vi "Labview_code_used_in_serum_and_PBS_experiments.vi"() -> ()   [LabVIEW 2018]
doc: "Example: Stream to Disk\n\nRecommended Input Signal: 100kHz, 2Vpp, sine wave\n\nDevices Supported: Refer to NI Example Finder\n\nLabVIEW Description:\n\nThis example demonstrates streaming a continuous acquisition to disk. It configures and starts one acquisition that is never triggered. This is accomplished by configuring a software trigger and never sending the software trigger. Therefore, the digitizer will continuously acquire data into its onboard memory until Abort or Close is called. \n\nThe loop continuously fetches data from onboard memory and streams it to a binary file. If the sampling rate is low, the computer can fetch all the data from the digitizer, so data is never overwritten. However, at faster sampling rates, the computer will not be able to fetch the data before it is overwritten by new data. This results in the \"data overwritten\" error.\n\nThe input parameters to the Fetch VI include the maximum waveform size to fetch. Since a timeout of zero is set, the digitizer will return however many points are currently available rather than waiting for the requested number of samples. The Fetch VI will return a waveform with the actual number of points fetched. \n\nThe \"relative to\" property determines which samples to fetch from memory. In this example, it is set to the read pointer, which starts at the beginning of the acquisition and is incremented by the actual number of points during each fetch."
uses:
  Interrogator design/Interrogator LABVIEW/2 cm/Control 1.ctl
  <vilib>/Utility/error.llb/DialogType.ctl
  <instrlib>/niScope/Controls/niScope input clock source.ctl
  <instrlib>/niScope/Controls/niScope exportable signals.ctl
  <instrlib>/niScope/Controls/niScope export destinations.ctl
  <instrlib>/niScope/Controls/niScope trigger source digital.ctl
  <instrlib>/niScope/Controls/niScope vertical coupling.ctl
  <vilib>/Analysis/3filter.llb/Filter Passband Type.ctl
  <vilib>/DAQmx/write.llb/DAQmx Write (Digital Wfm 1Chan NSamp).vi
  <vilib>/DAQmx/create/channels.llb/DAQmx Create Channel (DO-Digital Output).vi
  <vilib>/DAQmx/configure/timing.llb/DAQmx Timing (Sample Clock).vi
  <vilib>/DAQmx/configure/trigger.llb/DAQmx Start Trigger (Digital Edge).vi
  <vilib>/Waveform/DWDTOps.llb/DWDT Boolean Array to Digital.vi
  <vilib>/Waveform/DWDTOps.llb/DWDT Uncompress Digital.vi
  <vilib>/DAQmx/miscellaneous.llb/DAQmx Fill In Error Info.vi
  <instrlib>/niScope/Configure/Trigger/niScope Configure Trigger Digital.vi
  <instrlib>/niScope/Acquire/Fetch/niScope Fetch Binary 16.vi
  <vilib>/Analysis/3filter.llb/Butterworth Filter (DBL).vi
  <vilib>/measure/maresamp.llb/Resample Waveform (single shot).vi
  <vilib>/Analysis/3filter.llb/FIR Filter (DBL).vi
  <resource>/objmgr/daqmx.rc
  <vilib>/measure/NI_MAPro.lvlib
  <vilib>/Analysis/NI_AAL_SigProc.lvlib
  <vilib>/Analysis/NI_AALBase.lvlib
panel:
  out "element":i32
  out "Mod. depth":dbl
  out "Threshold 2":dbl
  out "Threshold 1":dbl
  out "Peak - Valley":dbl[](graph) caption="Peak - Valley vs. Sample Number"
  out "# of peaks":i32
  out "Resampled data":waveform(dbl)(graph) caption="Signal vs. Time"
  out "Peak det. output":bool[](array[boolean])
  in  "Sample rate":dbl=2000000.0 caption="Digital Output Frequency" step=1000000.0 format="%.3p"
  out "Acquisition Complete":bool=TRUE
  out "Digital Waveform":digitalwaveform(graph)
  in  "Line(s)":tag="PXI1Slot5/port0/line4"
  in  "stop":bool
  out "Total Acquired Data (bytes)":i64 format="%.0p"
  in  "Total Samples to Acquire":u64=10000000 step=1048576 format="%.3p"
  in  "Continues data acquisition":bool=TRUE caption="Plot Data?"
  out "Measurement Time (min)":dbl format="%.2f"
  out "Samples Used Onboard Memory":dbl(slide)=3898016.0 scale=-1.0..33554432.0 scale format="%.1p"
  out "Status":string="Acquisition in progress."
  out "Actual sample rate":dbl caption="Actual Sample Rate" format="%.3p"
  in  "Enforce realtime":bool=TRUE caption="Enforce Realtime"
  in  "Input Impedance":u32(ring) items=["1 mega ohm", "75 ohms", "50 ohms"]
  in  "Channel BW":T1=5000000.0 format="%.1p"
  in  "Channel":string="0" caption="Channel Name(s)"
  out "Format":string
  in  "Confirm File Replace?":bool
  in  "File path":path=path "C:/Users/trial.txt"
  out "error out":errorcluster {"code" format="%.0x"}
  out "Last Points Fetched":i32=50000 format="%.3p"
  out "Total Points Fetched":i64 format="%.0p"
  in  "resource name":refnum<k15>="PXI1Slot3" caption="Resource Name"
  in  "Max Points Per Fetch":u32=55000 format="%.3p"
  in  "Min sample rate":dbl=20000000.0 caption="Min Sample Rate" step=1000000.0 format="%.3p"
  in  "vertical range":dbl=2.5 caption="Vertical Range" format="%.2f"
  # "Vertical and Horizontal"
  # "Settings"
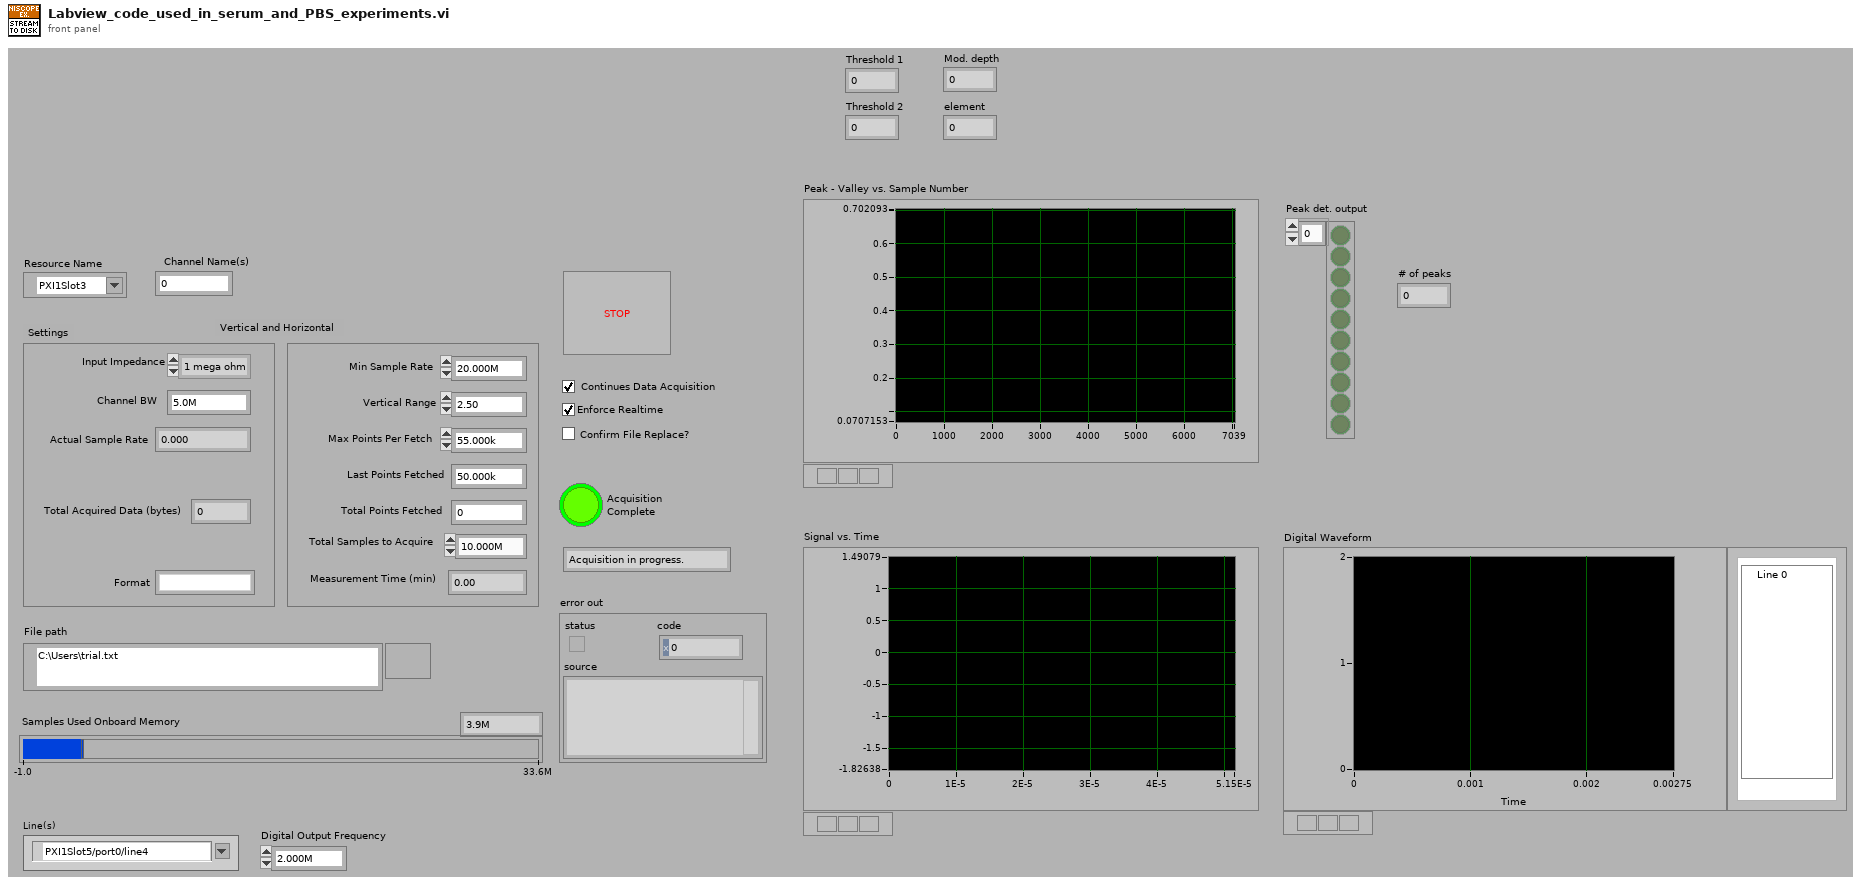
[diagram p1: front panel]
types:
  T1 = typedef "Control 1.ctl" = dbl
  T2 = typedef "niScope vertical coupling.ctl" = i32
  T3 = typedef "niScope trigger source digital.ctl" = string
  T4 = typedef "niScope export destinations.ctl" = string
  T5 = typedef "niScope exportable signals.ctl" = u16
  T6 = typedef "niScope input clock source.ctl" = u16
  T7 = typedef "DialogType.ctl" = u16
  T8 = enum16{"open", "open or create", "create or replace", "create", "open (read only)"}
  T9 = typedef "NI_AALBase.lvlib/Filter Passband Type.ctl" = enum32{"Lowpass", "Highpass", "Bandpass", "Bandstop"}
  T10 = cluster{"alias rejection (dB)":dbl, "normalized bandwidth":dbl}
  T11 = cluster{"actualSamples":i32, "absoluteInitialX":dbl, "relativeInitialX":dbl, "xIncrement":dbl, "offset":dbl, "gain":dbl, "reserved1":dbl, "reserved2":dbl}
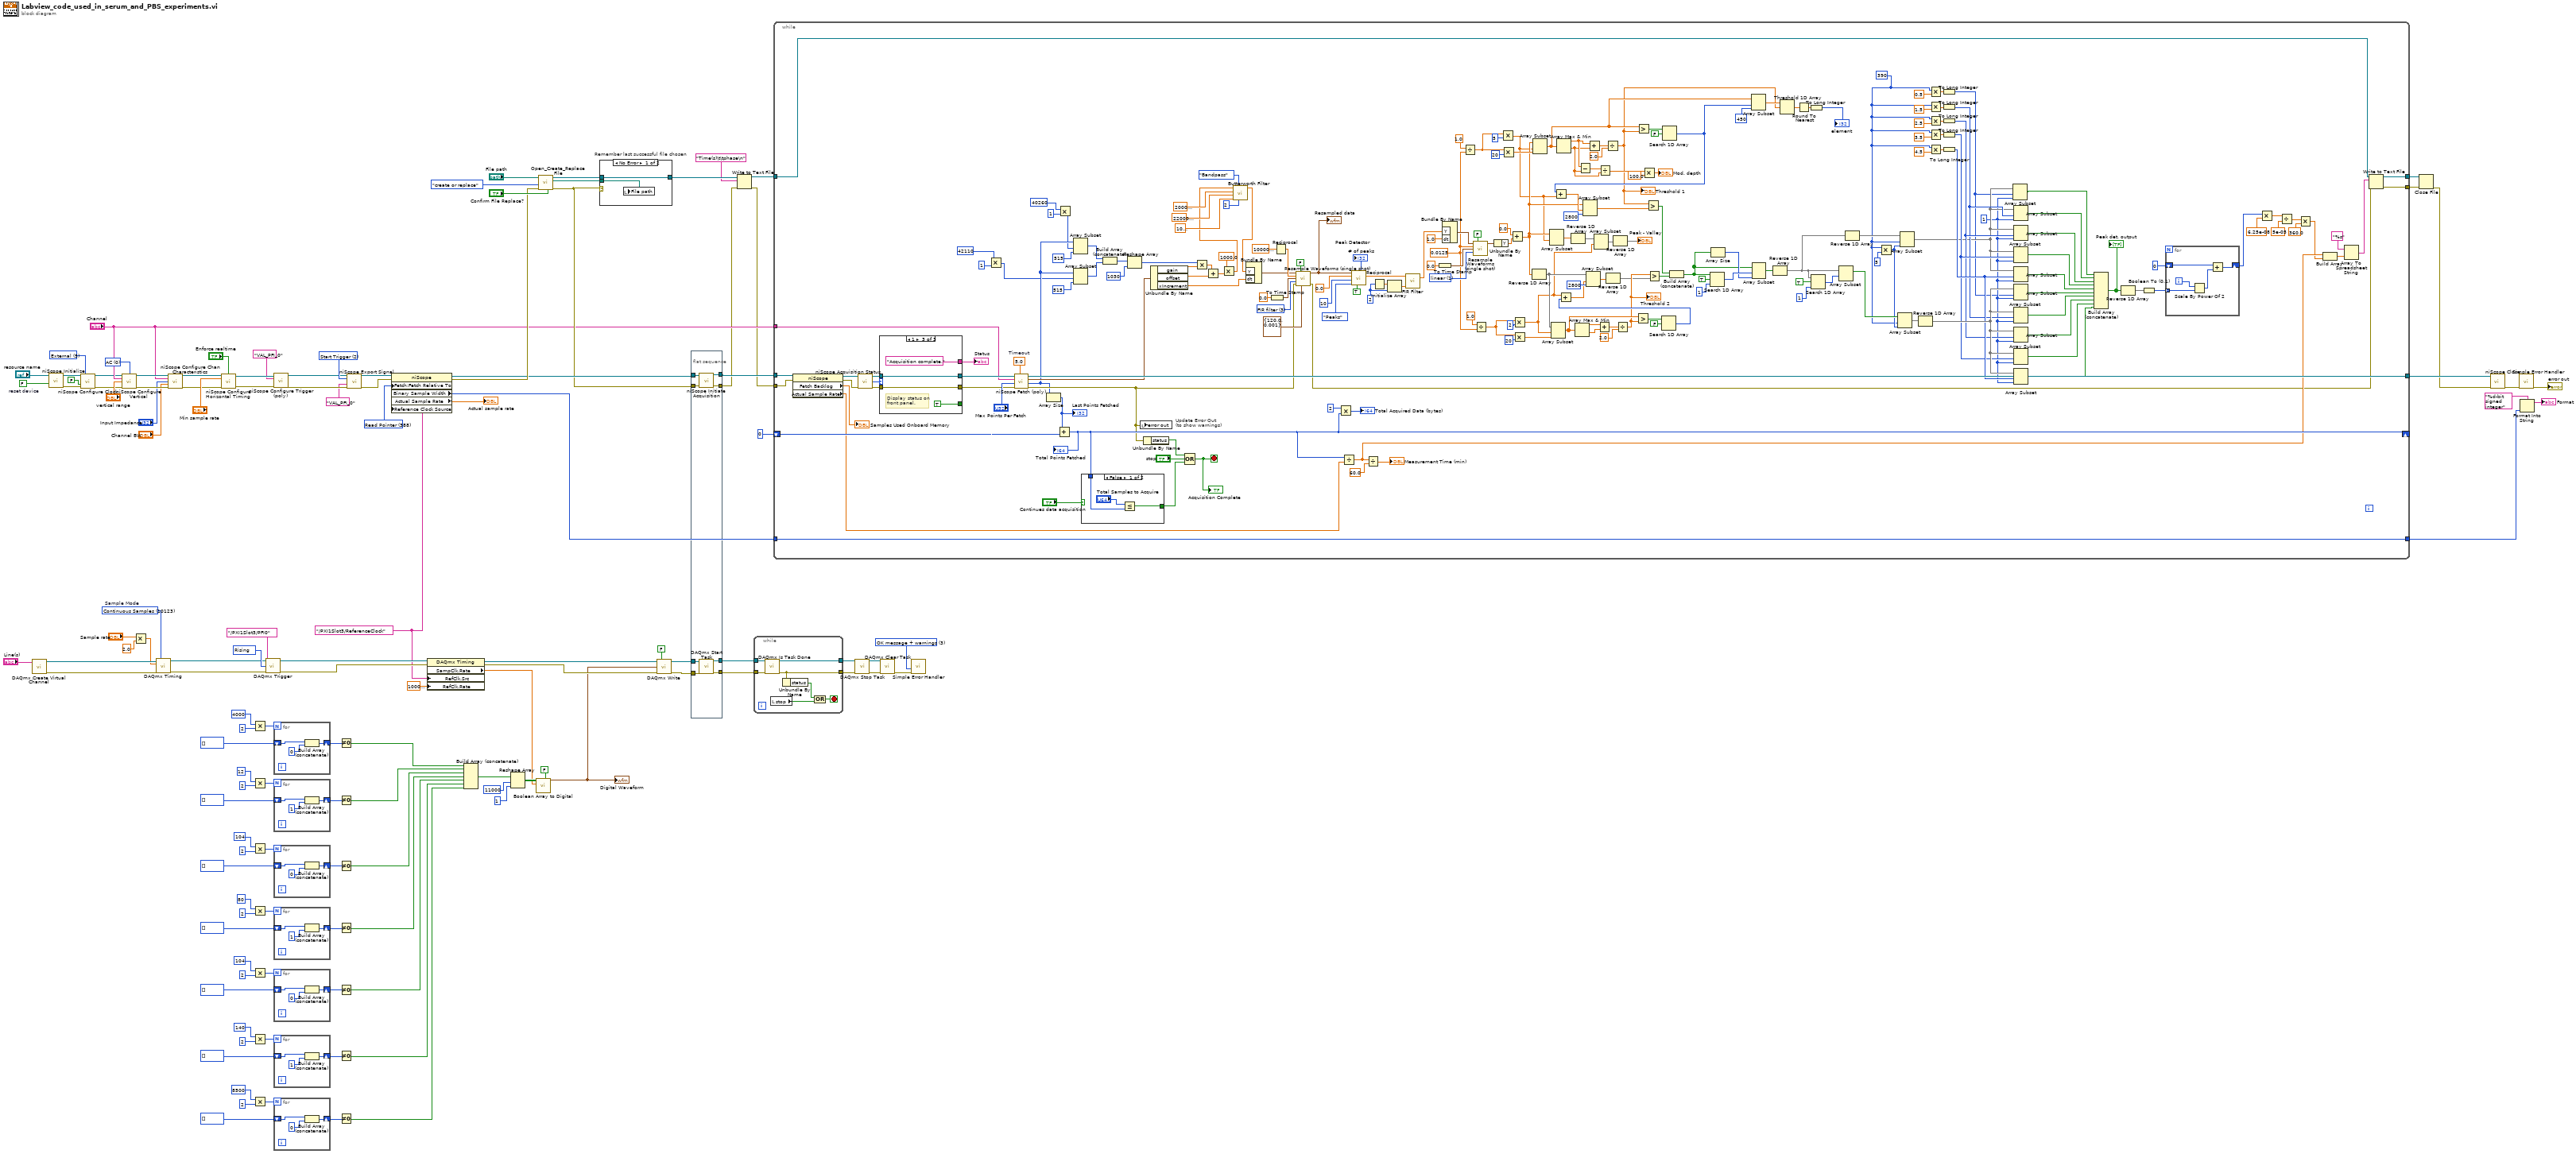
[diagram p0: block diagram]
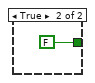
[diagram p3: hidden frame]
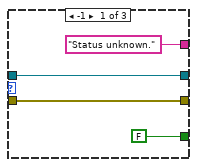
[diagram p4: hidden frame]
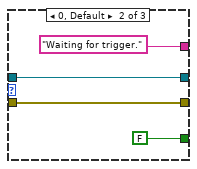
[diagram p5: hidden frame]
diagram:
  w1 = T2 0 items=["AC", "DC", "Ground"] ("vertical coupling")
  w3 = tag "/PXI1Slot3/ReferenceClock" ("source")
  w86 = 10280 items=["Rising"=10280, "Falling"=10171] ("edge")
  w91 = T5 2 items=["None"=0, "Start Trigger"=2, "Advance Trigger"=5, "Reference Trigger"=1, "End of Record Event"=4, "End of Acquisition Event"=3, "Ready for Start Event"=7, "Ready for Advance Event"=6, "Ready for Reference Event"=10, "Reference Clock"=100, "Sample Clock"=101, "5 Volt Power"=13] ("signal")
  w96 = 10123 items=["Finite Samples"=10178, "Continuous Samples"=10123, "Hardware Timed Single Point"=12522]  # Sample Mode
  w97 = T6 5 items=["None"=0, "RTSI Clock"=1, "PFI 0"=6, "PFI 1"=2, "PFI 2"=3, "PXI Clock"=4, "External"=5, "Clock In"=7] ("input clock source")
  w105 = T7 3 items=["no dialog", "OK message", "continue or stop message", "OK message + warnings", "continue/stop + warnings"] ("type of dialog (OK msg:1)")
  w114 = 388 items=["Start"=482, "Trigger"=483, "Pretrigger"=477, "Now"=481, "Read Pointer"=388] ("Fetch:Fetch Relative To")
  w132 = FALSE  # reset device
  # "Remember last successful file chosen"
  n1 = call-poly <vilib>:"DAQmx Create Virtual Channel.vi"("lines"="Line(s)") -> ("task out"=w57:refnum<k21>, "error out"=w56:errorcluster)  [unwired: 13 in]
  n2 = call <instrlib>:"niScope Initialize.vi"("resource name"="resource name", "reset device"=w132) -> ("instrument handle"=w104:refnum<k15>, "error out"=w103:errorcluster)  [unwired: 12 in]
  n3 = call <instrlib>:"niScope Configure Clock.vi"("instrument handle"=w104, "input clock source"=w97, "master enabled"=FALSE, "error in"=w103) -> ("instrument handle out"=w62:refnum<k15>, "error out"=w61:errorcluster)  [unwired: 10 in]
  n4 = call <instrlib>:"niScope Configure Vertical.vi"("instrument handle"=w62, "vertical coupling"=w1, "channels"="Channel", "vertical range"="vertical range", "error in"=w61) -> ("instrument handle out"=w119:refnum<k15>, "error out"=w118:errorcluster)  [unwired: 9 in]
  n5 = Multiply(x="Sample rate", y=2.0) -> (x*y=w54:dbl)
  n6 = call-poly <vilib>:"DAQmx Timing.vi"("task/channels in"=w57, "sample mode"=w96, "rate"=w54, "error in"=w56) -> ("task out"=w84:refnum<k21>, "error out"=w83:errorcluster)  [unwired: 10 in]
  n7 = call <instrlib>:"niScope Configure Chan Characteristics.vi"("instrument handle"=w119, "channels"="Channel", "input impedance"="Input Impedance", "maximum input frequency"="Channel BW", "error in"=w118) -> ("instrument handle out"=w59:refnum<k15>, "error out"=w58:errorcluster)  [unwired: 9 out]
  n8 = call <instrlib>:"niScope Configure Horizontal Timing.vi"("instrument handle"=w59, "enforce realtime"="Enforce realtime", "min sample rate"="Min sample rate", "error in"=w58) -> ("instrument handle out"=w89:refnum<k15>, "error out"=w88:errorcluster)  [unwired: 10 in]
  n9 = Multiply(x=4000, y=2) -> (x*y=w43:i32)
  n10 = Multiply(x=12, y=2) -> (x*y=w5:i32)
  n11 = Multiply(x=104, y=2) -> (x*y=w38:i32)
  n12 = Multiply(x=80, y=2) -> (x*y=w33:i32)
  n13 = Multiply(x=104, y=2) -> (x*y=w28:i32)
  n14 = Multiply(x=140, y=2) -> (x*y=w20:i32)
  n15 = Multiply(x=8500, y=2) -> (x*y=w13:i32)
  n16 = call-poly <vilib>:"DAQmx Trigger.vi"("task/channels in"=w84, "source"=tag "/PXI1Slot3/PFI0", "edge"=w86, "error in"=w83) -> ("task out"=w82:refnum<k21>, "error out"=w60:errorcluster)  [unwired: 10 in]
  n17 = call-poly <instrlib>:"niScope Configure Trigger (poly).vi"("instrument handle"=w89, "trigger source"=T3 "VAL_PFI_0", "error in"=w88) -> ("instrument handle out"=w72:refnum<k15>, "error out"=w92:errorcluster)  [unwired: 11 in]
  n18 = for {
    N: w43 -> [_]
    shift-right: [w133] -> w46
    shift-left: i32[] [] -> [w135]
    n19 = Build Array (concatenate)(w135, 0 ("element")) -> (w133:i32[])
  }
  n20 = for {
    N: w5 -> [_]
    shift-right: [w136] -> w8
    shift-left: i32[] [] -> [w138]
    n21 = Build Array (concatenate)(w138, 1 ("element")) -> (w136:i32[])
  }
  n22 = for {
    N: w38 -> [_]
    shift-right: [w139] -> w41
    shift-left: i32[] [] -> [w141]
    n23 = Build Array (concatenate)(w141, 0 ("element")) -> (w139:i32[])
  }
  n24 = for {
    N: w33 -> [_]
    shift-right: [w142] -> w36
    shift-left: i32[] [] -> [w144]
    n25 = Build Array (concatenate)(w144, 1 ("element")) -> (w142:i32[])
  }
  n26 = for {
    N: w28 -> [_]
    shift-right: [w145] -> w31
    shift-left: i32[] [] -> [w147]
    n27 = Build Array (concatenate)(w147, 0 ("element")) -> (w145:i32[])
  }
  n28 = for {
    N: w20 -> [_]
    shift-right: [w148] -> w22
    shift-left: i32[] [] -> [w150]
    n29 = Build Array (concatenate)(w150, 1 ("element")) -> (w148:i32[])
  }
  n30 = for {
    N: w13 -> [_]
    shift-right: [w151] -> w16
    shift-left: i32[] [] -> [w153]
    n31 = Build Array (concatenate)(w153, 0 ("element")) -> (w151:i32[])
  }
  n32 = Not Equal To 0?(x=w46) -> (x != 0?=w10:bool[])
  n33 = Not Equal To 0?(x=w8) -> (x != 0?=w4:bool[])
  n34 = Not Equal To 0?(x=w41) -> (x != 0?=w27:bool[])
  n35 = Not Equal To 0?(x=w36) -> (x != 0?=w25:bool[])
  n36 = Not Equal To 0?(x=w31) -> (x != 0?=w26:bool[])
  n37 = Not Equal To 0?(x=w22) -> (x != 0?=w18:bool[])
  n38 = Not Equal To 0?(x=w16) -> (x != 0?=w12:bool[])
  n39 = call <instrlib>:"niScope Export Signal.vi"("instrument handle"=w72, "signal"=w91, "output terminal"=T4 "VAL_PFI_0", "error in"=w92) -> ("instrument handle out"=w73:refnum<k15>, "error out"=w71:errorcluster)  [unwired: 10 in]
  n40 = property class="niScope"(reference=w73, error in=w71, "Fetch:Fetch Relative To"=w114, "Reference Clock Source"=w3) -> (reference out=w79:refnum<k15>, error out=w112:errorcluster, "Binary Sample Width"=w111:i32, "Actual Sample Rate"=→"Actual sample rate":dbl)
  n41 = property class="DAQmx Timing"(reference=w82, error in=w60, "RefClk.Src"=w3, "RefClk.Rate"=10000000.0 ("SampClk.Timebase.Rate")) -> (reference out=w81:refnum<k21>, error out=w80:errorcluster, "SampClk.Rate"=w24:dbl)
  n42 = Build Array (concatenate)(w10, w4, w27, w25, w26, w18, w12) -> (w50:bool[])
  n43 = Reshape Array(w50, 11000 ("dimension size"), 1 ("dimension size")) -> (w48:bool[][])
  n44 = call-poly <vilib>:"Boolean Array to Digital.vi"("compress data (F)"=FALSE, "sample rate"=w24, "boolean array"=w48) -> ("digital waveform"=w2:digitalwaveform)  [unwired: 7 in, 1 out]
  "Digital Waveform" <- w2
  n45 = call <vilib>:"Open_Create_Replace File.vi"("advisory dialog? (display:T)"="Confirm File Replace?", "error in (no error)"=w112, "function (open:0)"=T8."create or replace", "file path"="File path") -> ("error out"=w78:errorcluster, "new file path"=w127:path, "refnum"=w128:refnum<file>)  [unwired: 4 in, 1 out]
  n46 = case shown="No Error" w78 {
    tunnel: w127 -> [w154 _]
    tunnel: w128 -> [w155 w156]
    tunnel: [w155 w156] -> w68
    frame No Error {
      n47 = local write "File path"(w154) -> ()
    }
    frame Error {
    }
  }
  n48 = call-poly <vilib>:"DAQmx Write.vi"("task/channels in"=w81, "auto start"=FALSE, "data"=w2, "error in"=w80) -> ("task out"=w102:refnum<k21>, "error out"=w101:errorcluster)  [unwired: 9 in, 1 out]
  n49 = flat-sequence {
    tunnel: w102 -> [w164]
    tunnel: w101 -> [w163]
    tunnel: w79 -> [w160]
    tunnel: w78 -> [w159]
    tunnel: [w162] -> w70
    tunnel: [w161] -> w69
    tunnel: [w158] -> w77
    tunnel: [w157] -> w64
    frame #0 {
      n50 = call <instrlib>:"niScope Initiate Acquisition.vi"("instrument handle"=w160, "error in"=w159) -> ("instrument handle out"=w158:refnum<k15>, "error out"=w157:errorcluster)  [unwired: 12 in]
      n51 = call <vilib>:"DAQmx Start Task.vi"("task/channels in"=w164, "error in"=w163) -> ("task out"=w162:refnum<k21>, "error out"=w161:errorcluster)  [unwired: 12 in]
    }
  }
  n52 = Write to Text File(file (use dialog)=w68, text="Time(s)\t\tphase\n", error in=w64) -> (refnum out=w11:refnum<file>, error out=w63:errorcluster)  [unwired: 1 in, 1 out]
  n53 = while {
    tunnel: [w171] -> w100
    tunnel: [w170] -> w99
    tunnel: w70 -> [w166]
    tunnel: w69 -> [w165]
    stop <- w169 stop-if-true
    n54 = call <vilib>:"DAQmx Is Task Done.vi"("task/channels in"=w166, "error in"=w165) -> ("task out"=w171:refnum<k21>, "error out"=w170:errorcluster)  [unwired: 11 in, 1 out]
    n55 = local read "stop"() -> (w168:bool)
    n56 = Unbundle By Name(w170) -> ("status"=w167:bool)
    n57 = Compound Arithmetic op=OR(w167, w168) -> (w169:bool)
  }
  n58 = while {
    shift-left: 0 -> [w375]
    shift-right: [w355] -> _
    tunnel: "Channel" -> [w359]
    tunnel: w111 -> [w372]
    tunnel: [w372] -> w122
    tunnel: [w370] -> w120
    tunnel: w77 -> [w351]
    tunnel: w63 -> [w350]
    tunnel: [w331] -> w67
    tunnel: [w316] -> w65
    tunnel: w11 -> [w271]
    stop <- w348 stop-if-true
    w179 = 390 ("length")
    w228 = 2 ("x")
    w222 = 1 ("length")
    w306 = u16 1 items=["coerce", "linear", "spline", "FIR filter"] ("interpolation mode")
    w213 = 0.0125 ("dt")
    w327 = u16 3 items=["coerce", "linear", "spline", "FIR filter"] ("interpolation mode")
    w373 = 5.0  # Timeout
    # "Update Error Out\n(to show warnings)"
    n59 = property class="niScope"(reference=w351, error in=w350) -> (reference out=w320:refnum<k15>, error out=w352:errorcluster, "Fetch Backlog"=→"Samples Used Onboard Memory":dbl, "Actual Sample Rate"=w360:dbl)
    n60 = call <instrlib>:"niScope Acquisition Status.vi"("instrument handle"=w320, "error in"=w352) -> ("instrument handle out"=w367:refnum<k15>, "acquisition status"=w369:i32, "error out"=w368:errorcluster)  [unwired: 11 out]
    n61 = case shown="1" w369 {
      tunnel: w368 -> [w385 w390 w394]
      tunnel: w367 -> [w386 w391 w395]
      tunnel: ["Status unknown." "Waiting for trigger." "Acquisition complete."] -> w366
      tunnel: [w386 w391 w395] -> w364
      tunnel: [w385 w390 w394] -> w365
      tunnel: [FALSE ("value") FALSE ("value") TRUE ("value")] -> _
      frame -1 {
      }
      frame 0, Default {
      }
      frame 1 {
        # "Display status on\nfront panel."
      }
    }
    "Status" <- w366
    n62 = Multiply(x=42110 ("index"), y=1) -> (x*y=w277:i32)
    n63 = call-poly <instrlib>:"niScope Fetch (poly).vi"("timeout"=w373, "error in"=w365, "numSamples"="Max Points Per Fetch", "channels"=w359, "instrument handle"=w364) -> ("error out"=w317:errorcluster, "wfm"=w311:i16[], "wfm info"=w342:T11, "instrument handle out"=w370:refnum<k15>)  [unwired: 3 in]
    n64 = Array Size(array=w311) -> (size(s)=w371:i32)
    "Last Points Fetched" <- w371
    n65 = Add(x=w371, y=w375) -> (x+y=w355:i32)
    "Total Points Fetched" <- w355
    n66 = Multiply(x=40260 ("index"), y=1) -> (x*y=w280:i32)
    n67 = Array Subset(array=w311, index=w280, length=515) -> (w334:i16[])
    n68 = Array Subset(array=w311, index=w277, length=515) -> (w335:i16[])
    n69 = case shown="False" "Continues data acquisition" {
      tunnel: [w381 FALSE] -> w363
      tunnel: w355 -> [w382 _]
      frame False {
        n70 = Less Or Equal?(x="Total Samples to Acquire", y=w382) -> (x <= y?=w381:bool)
      }
      frame True {
      }
    }
    n71 = Build Array (concatenate)(w334, w335) -> (w333:i16[])
    n72 = Reshape Array(w333, 1030 ("dimension size")) -> (w310:i16[])
    n73 = local write "error out"(w317) -> ()
    n74 = Unbundle By Name(w317) -> ("status"=w349:bool)
    n75 = Unbundle By Name(w342) -> ("gain"=w345:dbl, "offset"=w346:dbl, "xIncrement"=w321:dbl)
    n76 = Compound Arithmetic op=OR(w349, "stop", w363) -> (w348:bool)
    "Acquisition Complete" <- w348
    n77 = Multiply(x=w310, y=w345) -> (x*y=w347:dbl[])
    n78 = Add(x=w347, y=w346) -> (x+y=w344:dbl[])
    n79 = Multiply(x=1000.0, y=w344) -> (x*y=w231:dbl[])
    n80 = call-poly <vilib>:"Butterworth Filter.vi"("order"=2, "filter type"=Filter_Passband_Type."Bandpass", "low cutoff freq: fl"=1000000.0, "high cutoff freq: fh"=2200000.0, "sampling freq: fs"=20000000.0, "X"=w231) -> ("Filtered X"=w230:dbl[])  [unwired: 2 in, 1 out]
    n81 = Bundle By Name("Y"=w230, "dt"=w321) -> (w275:waveform(dbl))  [unwired: 1 in]
    n82 = To Time Stamp(1:0.0 ("number")) -> (0:w324:timestamp)
    n83 = Reciprocal(x=100000000.0) -> (1/x=w326:dbl)
    n84 = call-poly <vilib>:"Resample Waveforms (single shot).vi"("waveform in"=w275, "open interval? (F)"=FALSE, "dt"=w326, "t0"=w324, "interpolation mode"=w327, "error in (no error)"=w317, "FIR filter specifications"=T10 {"alias rejection (dB)"=120.0, "normalized bandwidth"=0.001}) -> ("resampled waveform out"=w274:waveform(dbl), "error out"=w294:errorcluster)  [unwired: 5 in, 2 out]
    "Resampled data" <- w274
    n85 = Multiply(x=u64 2, y=w355) -> (x*y=→"Total Acquired Data (bytes)":u64)
    n86 = Divide(x=w355, y=w360) -> (x/y=w328:dbl)
    n87 = call <vilib>:"Peak Detector.vi"("initialize (T)"=TRUE, "peaks/valleys"=enum32{"Peaks", "Valleys"}."Peaks" ("peaks/valleys 2"), "width"=10, "threshold"=0.0, "X"=w274) -> ("Amplitudes"=w225:dbl[], "# found"=→"# of peaks":i32)  [unwired: 2 in, 3 out]
    n88 = Divide(x=w328, y=60.0) -> (x/y=→"Measurement Time (min)":dbl)
    n89 = Reciprocal(x=w228) -> (1/x=w229:dbl)
    n90 = Initialize Array(w229, w228) -> (w227:dbl[])
    n91 = call-poly <vilib>:"FIR Filter.vi"("FIR Coefficients"=w227, "X"=w225) -> ("Filtered X"=w226:dbl[])  [unwired: 2 in, 1 out]
    n92 = To Time Stamp(1:0.0 ("number")) -> (0:w304:timestamp)
    n93 = Bundle By Name("Y"=w226, "dt"=1.0) -> (w308:waveform(dbl))  [unwired: 1 in]
    n94 = Divide(x=1.0, y=w213) -> (x/y=w207:dbl)
    n95 = call-poly <vilib>:"Resample Waveforms (single shot).vi"("waveform in"=w308, "open interval? (F)"=FALSE, "dt"=w213, "t0"=w304, "interpolation mode"=w306) -> ("resampled waveform out"=w309:waveform(dbl))  [unwired: 7 in, 3 out]
    n96 = Divide(x=1.0, y=w213) -> (x/y=w205:dbl)
    n97 = Unbundle By Name(w309) -> ("Y"=w218:dbl[])
    n98 = Multiply(x=w207, y=5 ("length")) -> (x*y=w188:dbl)
    n99 = Multiply(x=w207, y=20 ("index")) -> (x*y=w215:dbl)
    n100 = Add(x=0.0, y=w218) -> (x+y=w189:dbl[])
    n101 = Multiply(x=w205, y=2 ("length")) -> (x*y=w185:dbl)
    n102 = Multiply(x=w205, y=20 ("index")) -> (x*y=w210:dbl)
    n103 = Reverse 1D Array(array=w189) -> (reversed array=w206:dbl[])
    n104 = Array Subset(array=w189, index=w188, length=w215) -> (w198:dbl[])
    n105 = Array Subset(array=w189, index=w188) -> (w187:dbl[])  [unwired: 1 in]
    n106 = Array Subset(array=w206, index=w185, length=w210) -> (w193:dbl[])
    n107 = Array Max & Min(array=w198) -> (max value=w242:dbl, min value=w240:dbl)  [unwired: 2 out]
    n108 = Reverse 1D Array(array=w187) -> (reversed array=w186:dbl[])
    n109 = Array Max & Min(array=w193) -> (max value=w264:dbl, min value=w265:dbl)  [unwired: 2 out]
    n110 = Subtract(x=w242, y=w240) -> (x-y=w241:dbl)
    n111 = Add(x=w242, y=w240) -> (x+y=w298:dbl)
    n112 = Array Subset(array=w186, index=w185) -> (w184:dbl[])  [unwired: 1 in]
    n113 = Add(x=w264, y=w265) -> (x+y=w267:dbl)
    n114 = Divide(x=w241, y=w240) -> (x/y=w239:dbl)
    n115 = Divide(x=w298, y=2.0) -> (x/y=w192:dbl)
    "Threshold 1" <- w192
    n116 = Reverse 1D Array(array=w184) -> (reversed array=→"Peak - Valley":dbl[])
    n117 = Divide(x=w267, y=2.0) -> (x/y=w190:dbl)
    "Threshold 2" <- w190
    n118 = Greater?(x=w193, y=w190) -> (0:w196:bool[])
    n119 = Greater?(x=w198, y=w192) -> (0:w200:bool[])
    n120 = Multiply(x=w239, y=100.0) -> (x*y=→"Mod. depth":dbl)
    n121 = Search 1D Array(1D array=w196, element=FALSE) -> (index of element=w194:i32)  [unwired: 1 in]
    n122 = Add(x=w185, y=w194) -> (x+y=w208:dbl)
    n123 = Array Subset(array=w206, index=w208, length=2800) -> (w204:dbl[])
    n124 = Reverse 1D Array(array=w204) -> (reversed array=w182:dbl[])
    n125 = Greater?(x=w190, y=w182) -> (0:w292:bool[])
    n126 = Search 1D Array(1D array=w200, element=FALSE) -> (index of element=w197:i32)  [unwired: 1 in]
    n127 = Add(x=w197, y=w188) -> (x+y=w209:dbl)
    n128 = Array Subset(array=w189, index=w209, length=2800) -> (w183:dbl[])
    n129 = Greater?(x=w192, y=w183) -> (0:w293:bool[])
    n130 = Build Array (concatenate)(w293, w292) -> (w191:bool[])
    n131 = Search 1D Array(1D array=w191, element=TRUE, start index (0)=1) -> (index of element=w340:i32)
    n132 = Array Size(array=w191) -> (size(s)=w302:i32)
    n133 = Array Subset(array=w198, index=w197, length=450) -> (w201:dbl[])
    n134 = Array Subset(array=w191, index=w340, length=w302) -> (w301:bool[])
    n135 = Reverse 1D Array(array=w301) -> (reversed array=w272:bool[])
    n136 = Threshold 1D Array(2:w192, 3:w201) -> (0:w203:dbl)  [unwired: 1 in]
    n137 = Round To Nearest(number=w203) -> (nearest integer value=w202:dbl)
    n138 = To Long Integer(number=w202) -> (32bit integer=→"element":i32)
    n139 = Search 1D Array(1D array=w272, element=TRUE, start index (0)=1) -> (index of element=w338:i32)
    n140 = Array Subset(array=w272, index=w338) -> (w273:bool[])  [unwired: 1 in]
    n141 = Reverse 1D Array(array=w272) -> (reversed array=w259:bool[])
    n142 = Multiply(x=w179, y=5) -> (x*y=w257:i32)
    n143 = Array Subset(array=w273, index=w179, length=w257) -> (w299:bool[])
    n144 = Array Subset(array=w259, index=w179, length=w257) -> (w223:bool[])
    n145 = Reverse 1D Array(array=w299) -> (reversed array=w276:bool[])
    n146 = Multiply(x=w179, y=0.5) -> (x*y=w249:dbl)
    n147 = Multiply(x=w179, y=1.5) -> (x*y=w255:dbl)
    n148 = Multiply(x=w179, y=2.5) -> (x*y=w253:dbl)
    n149 = Multiply(x=w179, y=3.5) -> (x*y=w251:dbl)
    n150 = Multiply(x=w179, y=4.5) -> (x*y=w247:dbl)
    n151 = To Long Integer(number=w249) -> (32bit integer=w221:i32)
    n152 = To Long Integer(number=w255) -> (32bit integer=w243:i32)
    n153 = To Long Integer(number=w253) -> (32bit integer=w244:i32)
    n154 = To Long Integer(number=w251) -> (32bit integer=w245:i32)
    n155 = To Long Integer(number=w247) -> (32bit integer=w246:i32)
    n156 = Array Subset(array=w223, index=w221, length=w222) -> (w224:bool[])
    n157 = Array Subset(array=w223, index=w243, length=w222) -> (w291:bool[])
    n158 = Array Subset(array=w223, index=w244, length=w222) -> (w290:bool[])
    n159 = Array Subset(array=w223, index=w245, length=w222) -> (w289:bool[])
    n160 = Array Subset(array=w223, index=w246, length=w222) -> (w288:bool[])
    n161 = Array Subset(array=w276, index=w221, length=w222) -> (w287:bool[])
    n162 = Array Subset(array=w276, index=w243, length=w222) -> (w286:bool[])
    n163 = Array Subset(array=w276, index=w244, length=w222) -> (w285:bool[])
    n164 = Array Subset(array=w276, index=w245, length=w222) -> (w284:bool[])
    n165 = Array Subset(array=w276, index=w246, length=w222) -> (w283:bool[])
    n166 = Build Array (concatenate)(w224, w291, w290, w289, w288, w287, w286, w285, w284, w283) -> (w262:bool[])
    "Peak det. output" <- w262
    n167 = Reverse 1D Array(array=w262) -> (reversed array=w263:bool[])
    n168 = Boolean To (0,1)(Boolean=w263) -> (0, 1=w261:i16[])
    n169 = for {
      tunnel: w261 -> [w379] mode=indexing
      shift-right: [w378] -> w173
      shift-left: i16 0 -> [w376]
      i -> [w380]
      n170 = Scale By Power Of 2(n=w380, x=w379) -> (x*2^n=w377:i16)
      n171 = Add(x=w376, y=w377) -> (x+y=w378:i16)
    }
    n172 = Multiply(x=w173, y=6.25e-08) -> (x*y=w177:dbl)
    n173 = Divide(x=w177, y=5e-05) -> (x/y=w175:dbl)
    n174 = Multiply(x=w175, y=360.0) -> (x*y=w172:dbl)
    n175 = Build Array(w328, w172) -> (w330:dbl[])
    n176 = Array To Spreadsheet String(array=w330, 3:"%s" ("format string")) -> (spreadsheet string=w318:string)  [unwired: 1 in]
    n177 = Write to Text File(file (use dialog)=w271, text=w318, error in=w294) -> (refnum out=w331:refnum<file>, error out=w316:errorcluster)  [unwired: 1 in, 1 out]
  }
  n178 = call <vilib>:"DAQmx Stop Task.vi"("task/channels in"=w100, "error in"=w99) -> ("task out"=w107:refnum<k21>, "error out"=w106:errorcluster)  [unwired: 12 in]
  n179 = call <vilib>:"DAQmx Clear Task.vi"("task in"=w107, "error in"=w106) -> ("error out"=w108:errorcluster)  [unwired: 13 in]
  n180 = call <vilib>:"Simple Error Handler.vi"("type of dialog (OK msg:1)"=w105, "error in (no error)"=w108) -> ()  [unwired: 3 in, 5 out]
  n181 = Close File(refnum=w67, error in=w65) -> (error out=w109:errorcluster)  [unwired: 1 out]
  n182 = call <instrlib>:"niScope Close.vi"("instrument handle"=w120, "error in"=w109) -> ("error out"=w110:errorcluster)  [unwired: 13 in]
  n183 = call <vilib>:"Simple Error Handler.vi"("error in (no error)"=w110) -> ("error out"=→"error out":errorcluster)  [unwired: 4 in, 4 out]
  n184 = Format Into String(format string="%d-bit signed integer", w122) -> (resulting string=→"Format":string)  [unwired: 2 in, 1 out]
